vi "Measurement Parser.vi"(8 "error in (no error)":errorcluster, 9 "Generic Instrument.lvlib:Generic Card.lvclass":refnum<class "Generic Card.lvclass">, 10 "Data Array":dbl[](array[numeric]), 11 "Yokogawa WT2X0 in":refnum<class "Yokogawa WT2X0.lvclass">) -> (0 "error out":errorcluster, 2 "Waveform Graph":dynamicdata(graph), 3 "Yokogawa WT2X0 out":refnum<class "Yokogawa WT2X0.lvclass">)   [LabVIEW 2014, in "Generic Power Analyzer.lvlib" / "Yokogawa WT2X0.lvlib" / "Yokogawa WT2X0.lvclass"]
uses:
  Yokogawa WT2X0.lvclass
  Generic Instrument/Generic Card/Generic Card.lvclass
  Generic Instrument/Generic Card/Generic Card.lvclass/Generic Card.ctl
  Data Logger/Data Logger.lvclass
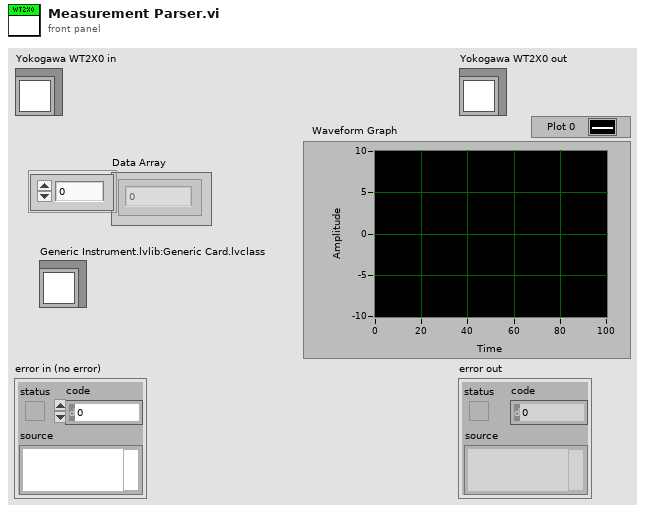
[diagram p1: front panel]
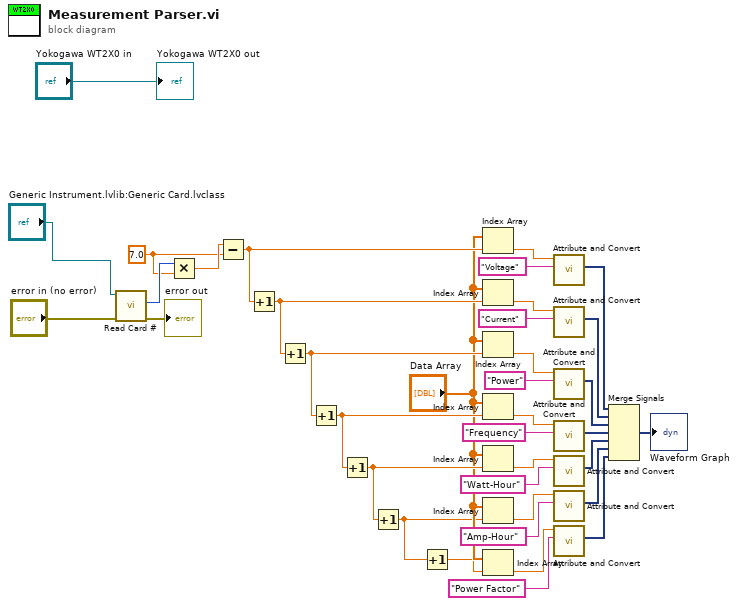
[diagram p0: block diagram]
diagram:
  w35 = 7.0 ("y")
  n1 = call "Read Card #.vi"("error in (no error)"="error in (no error)", "Generic Card in"="Generic Instrument.lvlib:Generic Card.lvclass") -> ("error out"=→"error out":errorcluster, "Card #"=w37:u8)  [unwired: 7 in, 1 out]
  n2 = Multiply(x=w37, y=w35) -> (x*y=w36:dbl)
  n3 = Subtract(x=w36, y=w35) -> (x-y=w24:dbl)
  n4 = Increment(x=w24) -> (x+1=w23:dbl)
  n5 = Increment(x=w23) -> (x+1=w21:dbl)
  n6 = Increment(x=w21) -> (x+1=w19:dbl)
  n7 = Increment(x=w19) -> (x+1=w17:dbl)
  n8 = Increment(x=w17) -> (x+1=w3:dbl)
  n9 = Increment(x=w3) -> (x+1=w2:dbl)
  n10 = Index Array(array="Data Array", index=w24) -> (element=w34:dbl)
  n11 = Index Array(array="Data Array", index=w23) -> (element=w25:dbl)
  n12 = Index Array(array="Data Array", index=w21) -> (element=w22:dbl)
  n13 = Index Array(array="Data Array", index=w19) -> (element=w20:dbl)
  n14 = Index Array(array="Data Array", index=w17) -> (element=w18:dbl)
  n15 = Index Array(array="Data Array", index=w3) -> (element=w16:dbl)
  n16 = Index Array(array="Data Array", index=w2) -> (element=w6:dbl)
  n17 = call "Attribute and Convert.vi"("Signal Name"="Voltage", "Number in"=w34) -> ("Dynamic Signal Out"=w15:dynamicdata)  [unwired: 9 in]
  n18 = call "Attribute and Convert.vi"("Signal Name"="Current", "Number in"=w25) -> ("Dynamic Signal Out"=w14:dynamicdata)  [unwired: 9 in]
  n19 = call "Attribute and Convert.vi"("Signal Name"="Power", "Number in"=w22) -> ("Dynamic Signal Out"=w13:dynamicdata)  [unwired: 9 in]
  n20 = call "Attribute and Convert.vi"("Signal Name"="Frequency", "Number in"=w20) -> ("Dynamic Signal Out"=w12:dynamicdata)  [unwired: 9 in]
  n21 = call "Attribute and Convert.vi"("Signal Name"="Watt-Hour", "Number in"=w18) -> ("Dynamic Signal Out"=w11:dynamicdata)  [unwired: 9 in]
  n22 = call "Attribute and Convert.vi"("Signal Name"="Amp-Hour", "Number in"=w16) -> ("Dynamic Signal Out"=w10:dynamicdata)  [unwired: 9 in]
  n23 = call "Attribute and Convert.vi"("Signal Name"="Power Factor", "Number in"=w6) -> ("Dynamic Signal Out"=w4:dynamicdata)  [unwired: 9 in]
  n24 = Merge Signals(w15, w14, w13, w12, w11, w10, w4) -> (→"Waveform Graph":dynamicdata)
  "Yokogawa WT2X0 out" <- "Yokogawa WT2X0 in"
